vi "fft -- waveform manipulate -- V1.vi"(6 "time (sec)":dbl=-0.01 format="%#_3p", 7 "fft -- manipulate":T1, 8 "Map IN":map{dbl, dbl}(c390), 9 "Ref Cluster IN":cluster{dbl[], dbl[]}, 10 "Cluster IN":cluster{dbl[], dbl[]}, 11 "Waveform IN":waveform(dbl)) -> (0 "Map out":map{dbl, dbl}(c390), 1 "Ref Cluster OUT":cluster{dbl[], dbl[]}, 2 "Cluster out":cluster{dbl[], dbl[]}, 3 "Waveform OUT":waveform(dbl))   [LabVIEW 2021]
uses:
  fft -- waveform manipulate -- control.vi.ctl
  <vilib>/gmath/NI_Gmath.lvlib
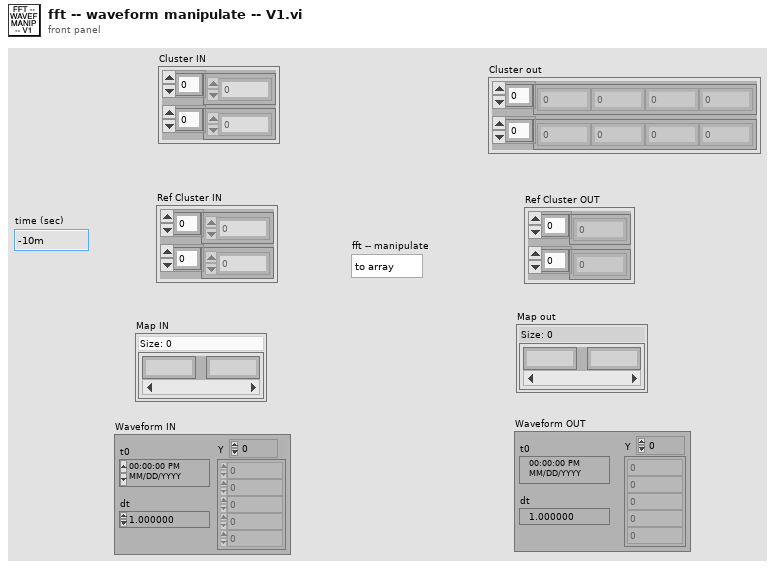
[diagram p1: front panel]
types:
  T1 = typedef "fft -- waveform manipulate -- control.vi.ctl" = enum16{"to array", "to map", "ref from map", "interp from map", "interp from array", "interp other", "delay"}
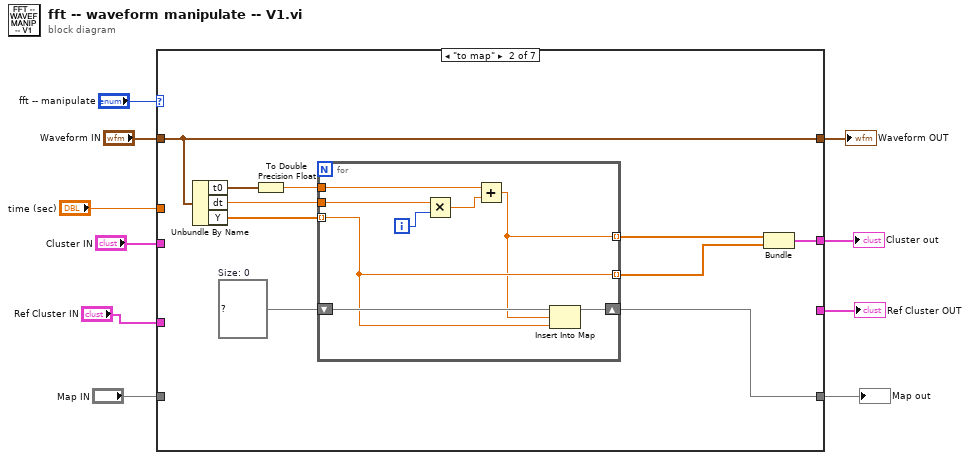
[diagram p0: block diagram]
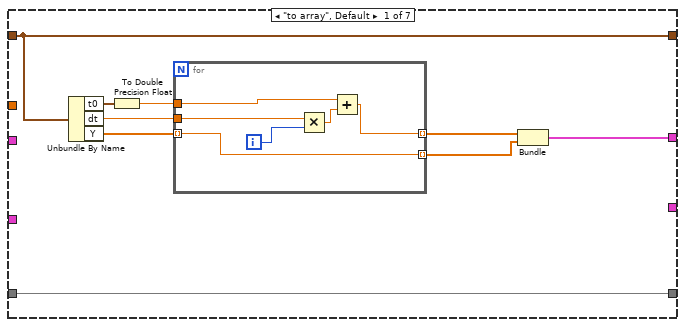
[diagram p2: hidden frame]
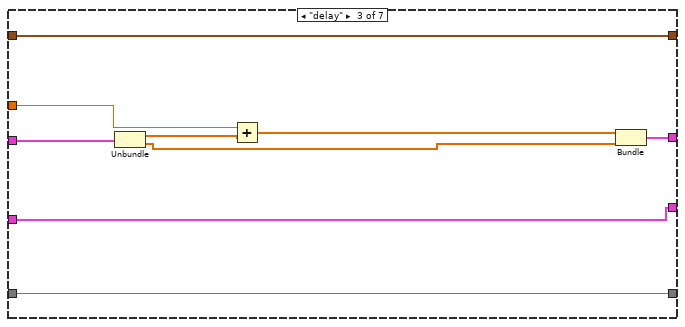
[diagram p3: hidden frame]
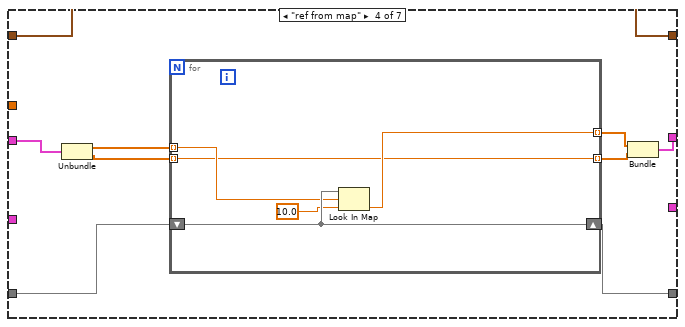
[diagram p4: hidden frame]
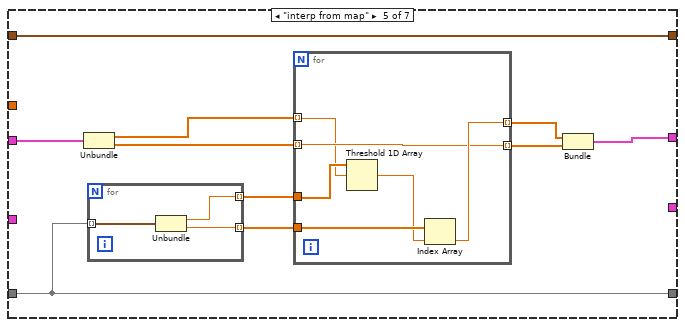
[diagram p5: hidden frame]
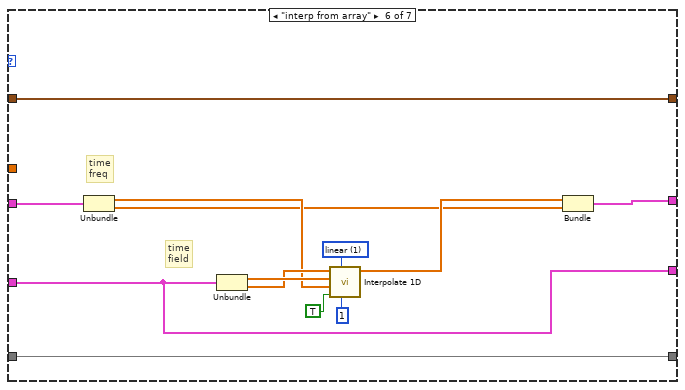
[diagram p6: hidden frame]
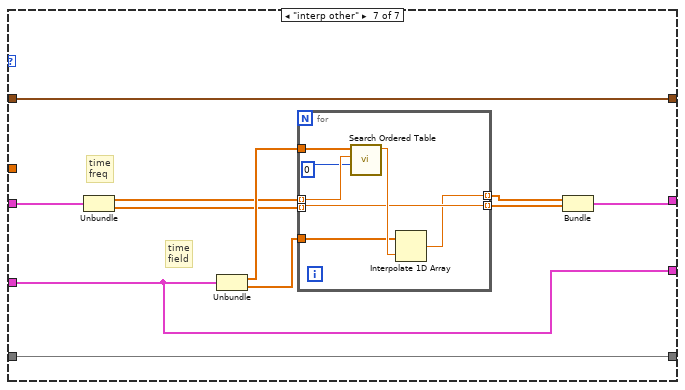
[diagram p7: hidden frame]
diagram:
  n1 = case shown="\"to map\"" "fft -- manipulate" {
    tunnel: "Waveform IN" -> [w14 w29 w52 w55 w76 w98 w109]
    tunnel: [w13 w30 w51 w61 w68 w96 w107] -> w8
    tunnel: "Map IN" -> [w13 _ w51 w60 w68 w96 w107]
    tunnel: [w15 w26 w45 w56 w69 w87 w99] -> w6
    tunnel: [w14 w29 w52 w55 w76 w98 w109] -> w5
    tunnel: "Cluster IN" -> [_ _ w50 w59 w75 w97 w108]
    tunnel: "Ref Cluster IN" -> [_ _ w44 _ _ w86 w106]
    tunnel: [_ _ w44 _ _ w86 w106] -> w2
    tunnel: "time (sec)" -> [_ _ w48 _ _ _ _]
    frame "to array", Default {
      n2 = Unbundle By Name(w14) -> ("t0"=w17:timestamp, "dt"=w19:dbl, "Y"=w18:dbl[])
      n3 = To Double Precision Float(number=w17) -> (double precision float=w16:dbl)
      n4 = for {
        tunnel: w19 -> [w23]
        tunnel: w16 -> [w22]
        tunnel: w18 -> [w20] mode=indexing
        tunnel: [w21] -> w12 mode=indexing
        tunnel: [w20] -> w11 mode=indexing
        i -> [w25]
        n5 = Multiply(x=w23, y=w25) -> (x*y=w24:dbl)
        n6 = Add(x=w22, y=w24) -> (x+y=w21:dbl)
      }
      n7 = Bundle(w12, w11) -> (w15:cluster{dbl[], dbl[]})  [unwired: 1 in]
    }
    frame "to map" {
      w35 = map{dbl, dbl} {}  # Size: 0
      n8 = Unbundle By Name(w29) -> ("t0"=w32:timestamp, "dt"=w34:dbl, "Y"=w33:dbl[])
      n9 = To Double Precision Float(number=w32) -> (double precision float=w31:dbl)
      n10 = for {
        shift-right: [w38] -> w30
        shift-left: w35 -> [w39]
        tunnel: w34 -> [w41]
        tunnel: w31 -> [w40]
        tunnel: w33 -> [w37] mode=indexing
        tunnel: [w37] -> w27 mode=indexing
        tunnel: [w36] -> w28 mode=indexing
        i -> [w43]
        n11 = Multiply(x=w41, y=w43) -> (x*y=w42:dbl)
        n12 = Add(x=w40, y=w42) -> (x+y=w36:dbl)
        n13 = Insert Into Map(map in=w39, key=w36, value=w37) -> (map out=w38:map{dbl, dbl})  [unwired: 2 out]
      }
      n14 = Bundle(w28, w27) -> (w26:cluster{dbl[], dbl[]})  [unwired: 1 in]
    }
    frame "delay" {
      n15 = Unbundle(w50) -> (w49:dbl[], w47:dbl[])
      n16 = Add(x=w48, y=w49) -> (x+y=w46:dbl[])
      n17 = Bundle(w46, w47) -> (w45:cluster{dbl[], dbl[]})  [unwired: 1 in]
    }
    frame "ref from map" {
      n18 = Unbundle(w59) -> (w58:dbl[], w57:dbl[])
      n19 = for {
        shift-right: [w66] -> w61
        shift-left: w60 -> [w66]
        tunnel: w58 -> [w65] mode=indexing
        tunnel: w57 -> [w63] mode=indexing
        tunnel: [w64] -> w54 mode=indexing
        tunnel: [w63] -> w53 mode=indexing
        n20 = Look In Map(map=w66, key=w65, default value=10.0) -> (value=w64:dbl)  [unwired: 1 out]
      }
      n21 = Bundle(w54, w53) -> (w56:cluster{dbl[], dbl[]})  [unwired: 1 in]
    }
    frame "interp from map" {
      n22 = Unbundle(w75) -> (w74:dbl[], w72:dbl[])
      n23 = for {
        tunnel: w68 -> [w79] mode=indexing
        tunnel: [w78] -> w67 mode=indexing
        tunnel: [w77] -> w73 mode=indexing
        n24 = Unbundle(w79) -> ("dt"=w78:dbl, w77:dbl)
      }
      n25 = for {
        tunnel: w74 -> [w81] mode=indexing
        tunnel: w73 -> [w85]
        tunnel: [w84] -> w71 mode=indexing
        tunnel: [w83] -> w70 mode=indexing
        tunnel: w72 -> [w83] mode=indexing
        tunnel: w67 -> [w82]
        n26 = Threshold 1D Array(2:w81, 3:w82) -> (0:w80:dbl)  [unwired: 1 in]
        n27 = Index Array(array=w85, index=w80) -> (element=w84:dbl)
      }
      n28 = Bundle(w71, w70) -> (w69:cluster{dbl[], dbl[]})  [unwired: 1 in]
    }
    frame "interp from array" {
      w95 = 1 items=["nearest", "linear", "spline", "cubic Hermite", "Lagrange"] ("method")
      # "time\nfield"
      # "time\nfreq"
      n29 = Unbundle(w97) -> (w90:dbl[], w88:dbl[])
      n30 = Unbundle(w86) -> (w92:dbl[], w91:dbl[])
      n31 = call <vilib>:"Interpolate 1D.vi"("ntimes"=1, "method"=w95, "X is monotonic"=TRUE, "xi"=w90, "X"=w92, "Y"=w91) -> ("yi"=w89:dbl[])  [unwired: 3 in, 2 out]
      n32 = Bundle("yi"=w89, w88) -> (w87:cluster{"yi":dbl[], dbl[]})  [unwired: 1 in]
    }
    frame "interp other" {
      # "time\nfield"
      # "time\nfreq"
      n33 = Unbundle(w108) -> (w104:dbl[], w102:dbl[])
      n34 = Unbundle(w106) -> (w105:dbl[], w103:dbl[])
      n35 = for {
        tunnel: w105 -> [w116]
        tunnel: w104 -> [w115] mode=indexing
        tunnel: w103 -> [w112]
        tunnel: w102 -> [w111] mode=indexing
        tunnel: [w111] -> w101 mode=indexing
        tunnel: [w110] -> w100 mode=indexing
        n36 = call <vilib>:"Search Ordered Table.vi"("starting index"=0, "x value"=w115, "ordered x array"=w116) -> ("fractional index"=w113:dbl)  [unwired: 8 in]
        n37 = Interpolate 1D Array(1:w113, 2:w112) -> (0:w110:dbl)
      }
      n38 = Bundle(w100, w101) -> (w99:cluster{dbl[], dbl[]})  [unwired: 1 in]
    }
  }
  "Map out" <- w8
  "Cluster out" <- w6
  "Waveform OUT" <- w5
  "Ref Cluster OUT" <- w2
